vi "Calculate Iterations and Array Size.vi"(9 "Updates per Second":dbl, 10 "Loop Period":dbl, 11 "Time in Seconds":dbl) -> (1 "Loop Duration (s)":dbl, 2 "Generated Numbers per Iteration":i32, 3 "Loop Iterations":i32)   [LabVIEW 2020, in "UIProgressUpdates.lvlib"]
uses:
  UIProgressUpdates.lvlib
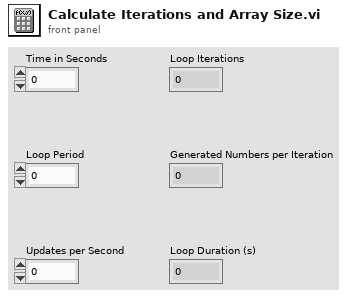
[diagram p1: front panel]
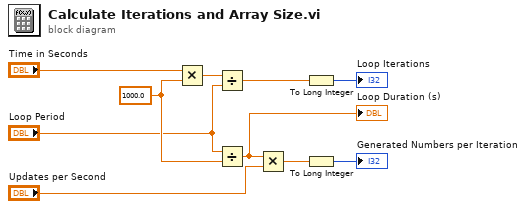
[diagram p0: block diagram]
diagram:
  w3 = 1000.0 ("y")
  n1 = Multiply(x="Time in Seconds", y=w3) -> (x*y=w5:dbl)
  n2 = Divide(x=w5, y="Loop Period") -> (x/y=w6:dbl)
  n3 = Divide(x="Loop Period", y=w3) -> (x/y=w1:dbl)
  "Loop Duration (s)" <- w1
  n4 = Multiply(x=w1, y="Updates per Second") -> (x*y=w9:dbl)
  n5 = To Long Integer(number=w6) -> (32bit integer=→"Loop Iterations":i32)
  n6 = To Long Integer(number=w9) -> (32bit integer=→"Generated Numbers per Iteration":i32)
